vi "NIIE_DoubleClick.vi"(7 "Fill Color":T7=16860, 8 "Error":errorcluster, 9 "Data":T1={"Class"={"Ants"=refnum, "Layer"=refnum, "Templates"=refnum, "Icon"=refnum, "Glyph"=refnum, "Settings"=refnum, "Tools"=refnum}, "Ref"={"Add Layer"=refnum, "Remove Layer"=refnum, "Line Text"=[], "Body Text Spec"=refnum, "DNL_Font"=refnum, "glyph path str"=refnum, "templates path str"=refnum, "Arrow Up"=refnum, "Arrow Down"=refnum, "IE VI Ref"=refnum, "Glyphs tree"=refnum, "Templates tree"=refnum, "Layer Icon Text"=refnum, "Layer Template"=refnum, "Clipboard"=refnum, "BW icon in"=refnum, "Color icon in"=refnum, "Layer Clust"=refnum, "Body Text"=refnum, "DNL_Framework Templates"=refnum, "Search Templates"=refnum, "TextMarker"=refnum, "Tab Control"=refnum, "Search Glyphs"=refnum, "Line Color"=refnum, "DNL_Glyphs []"=refnum, "Fill Color"=refnum, "Tools"=refnum, "Glyphs tree"=refnum, "Icon"=refnum, "Preview"=refnum, "Ants"=refnum, "Terminals"=refnum, "menu reference"=refnum, "LayerNames"=[], "GlyphLoadAnimation"=refnum, "TemplateLoadAnimation"=refnum, "refreshGlyphs"=refnum, "refreshTemplates"=refnum}, "Support"={"AntsRect"={"left"=0, "top"=0, "right"=0, "bottom"=0}, "Mouse Move Coords"={"Horizontal"=0, "Vertical"=0}, "Mouse Down Coords"={"Horizontal"=0, "Vertical"=0}, "Temp Coord"={"Horizontal"=0, "Vertical"=0}, "Action"=enum."Default", "Edge Color"=4914962, "Fill Color"=16860, "Mouse Down?"=FALSE, "Draft Mode?"=FALSE, "Temp Icon"=bytes[3102], "CTRL Pressed"=FALSE, "Move Selection?"=FALSE, "AntsRect Orig"={"left"=0, "top"=0, "right"=0, "bottom"=0}, "Text"="", "TM Set?"=FALSE, "Mouse inside icon?"=FALSE, "Tool (old value)"=0, "Pencil Move Color"=0, "Swap Colors?"=FALSE, "Shift pressed?"=FALSE}}, 11 "Edge Color":T7=16860) -> (0 "Error Out":errorcluster, 1 "Name Out":string, 3 "New Picture Out":picture, 4 "Active Tool Out":T8=enum."Ellipse", 5 "Invalid Picture? Out":bool)   [LabVIEW 2021]
uses:
  vi.lib/LabVIEW Icon API/lv_icon/Controls/IEColor.ctl
  MB CORE/TypeDefs/Cluster_Button Draw Tools.ctl
  MB CORE/TypeDefs/Bool_Draw Tool.ctl
  MB CORE/TypeDefs/Bool_Line Tool.ctl
  MB CORE/TypeDefs/Bool_ColorExtractor Tool.ctl
  MB CORE/TypeDefs/Bool_Fill Tool.ctl
  MB CORE/TypeDefs/Bool_IERect Tool.ctl
  MB CORE/TypeDefs/Bool_FRect Tool.ctl
  MB CORE/TypeDefs/Bool_Circle Tool.ctl
  MB CORE/TypeDefs/Bool_FillCircle Tool.ctl
  MB CORE/TypeDefs/Bool_Eraser Tool.ctl
  MB CORE/TypeDefs/Bool_Text Tool.ctl
  MB CORE/TypeDefs/Bool_Selection Tool.ctl
  MB CORE/TypeDefs/Bool_Move Tool.ctl
  Controls/IE Data.ctl
  Class/Tools/Tools Paint.lvclass
  Class/Ants/Ants.lvclass
  Class/FakedArray/FakedArray.lvclass
  vi.lib/LabVIEW Icon API/lv_icon/Classes/Icon/Icon.lvclass
  Class/Icon Library/Glyph.lvclass
  Class/Settings/Settings.lvclass
  Controls/IE Classes.ctl
  Controls/References Cluster.ctl
  Controls/SupportClass.ctl
  <vilib>/Utility/miscctls.llb/LVPoint32TypeDef.ctl
  Controls/ENUM_SupportClass_Action.ctl
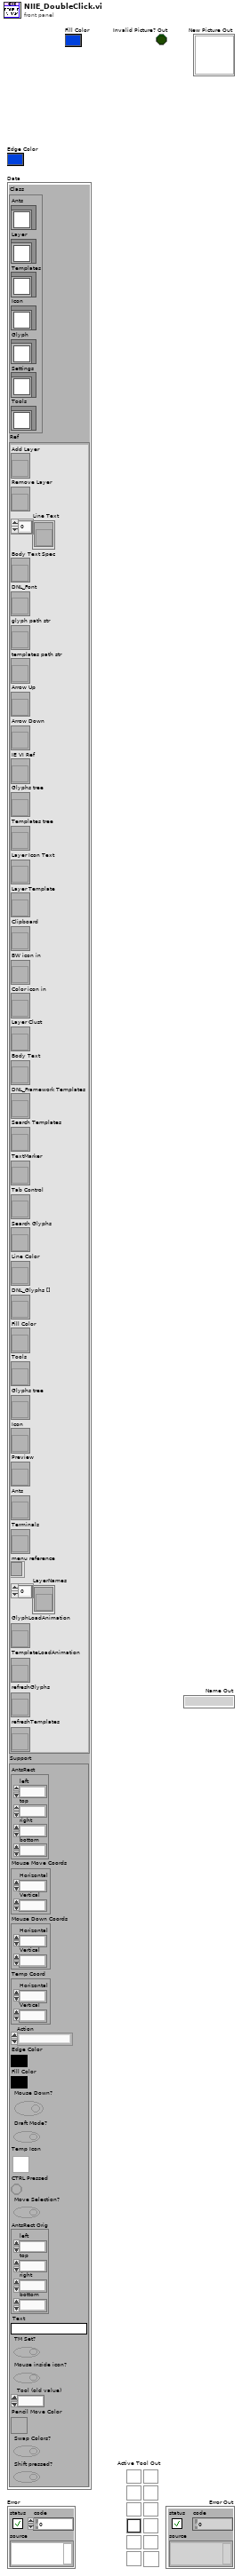
[diagram p1: front panel]
types:
  T1 = typedef "IE Data.ctl" = cluster{"Class":T2, "Ref":T3, "Support":T4}
  T2 = typedef "IE Classes.ctl" = cluster{"Ants":refnum<class "Ants.lvclass">, "Layer":refnum<class "FakedArray.lvclass">, "Templates":refnum<class "FakedArray.lvclass">, "Icon":refnum<class "Icon.lvclass">, "Glyph":refnum<class "Glyph.lvclass">, "Settings":refnum<class "Settings.lvclass">, "Tools":refnum<class "Tools Paint.lvclass">}
  T3 = typedef "References Cluster.ctl" = cluster{"Add Layer":refnum<vi>, "Remove Layer":refnum<vi>, "Line Text":refnum<vi>[], "Body Text Spec":refnum<vi>, "DNL_Font":refnum<vi>, "glyph path str":refnum<vi>, "templates path str":refnum<vi>, "Arrow Up":refnum<vi>, "Arrow Down":refnum<vi>, "IE VI Ref":refnum<vi>, "Glyphs tree":refnum<vi>, "Templates tree":refnum<vi>, "Layer Icon Text":refnum<vi>, "Layer Template":refnum<vi>, "Clipboard":refnum<vi>, "BW icon in":refnum<vi>, "Color icon in":refnum<vi>, "Layer Clust":refnum<vi>, "Body Text":refnum<vi>, "DNL_Framework Templates":refnum<vi>, "Search Templates":refnum<vi>, "TextMarker":refnum<vi>, "Tab Control":refnum<vi>, "Search Glyphs":refnum<vi>, "Line Color":refnum<vi>, "DNL_Glyphs []":refnum<vi>, "Fill Color":refnum<vi>, "Tools":refnum<vi>, "Glyphs tree":refnum<vi>, "Icon":refnum<vi>, "Preview":refnum<vi>, "Ants":refnum<vi>, "Terminals":refnum<vi>, "menu reference":refnum<k9>, "LayerNames":refnum<vi>[], "GlyphLoadAnimation":refnum<vi>, "TemplateLoadAnimation":refnum<vi>, "refreshGlyphs":refnum<vi>, "refreshTemplates":refnum<vi>}
  T4 = typedef "SupportClass.ctl" = cluster{"AntsRect":cluster{"left":i16, "top":i16, "right":i16, "bottom":i16}, "Mouse Move Coords":T5, "Mouse Down Coords":T5, "Temp Coord":T5, "Action":T6, "Edge Color":T7, "Fill Color":T7, "Mouse Down?":bool, "Draft Mode?":bool, "Temp Icon":picture, "CTRL Pressed":bool, "Move Selection?":bool, "AntsRect Orig":cluster{"left":i16, "top":i16, "right":i16, "bottom":i16}, "Text":string, "TM Set?":bool, "Mouse inside icon?":bool, "Tool (old value)":u32, "Pencil Move Color":u32, "Swap Colors?":bool, "Shift pressed?":bool}
  T5 = typedef "LVPoint32TypeDef.ctl" = cluster{"Horizontal":i32, "Vertical":i32}
  T6 = typedef "ENUM_SupportClass_Action.ctl" = enum16{"Default", "Move Selection", "Glyph Library", "Tool"}
  T7 = typedef "IEColor.ctl" = u32
  T8 = typedef "Cluster_Button Draw Tools.ctl" = enum32{"Pencil", "Line", "Dropper", "Fill", "Rectangle", "Filled Rectangle", "Ellipse", "Filled Ellipse", "Eraser", "Text", "Select", "Move"}
  T9 = cluster{"left":i16, "top":i16, "right":i16, "bottom":i16}
  T10 = cluster{"Left":i32, "Top":i32, "Right":i32, "Bottom":i32}
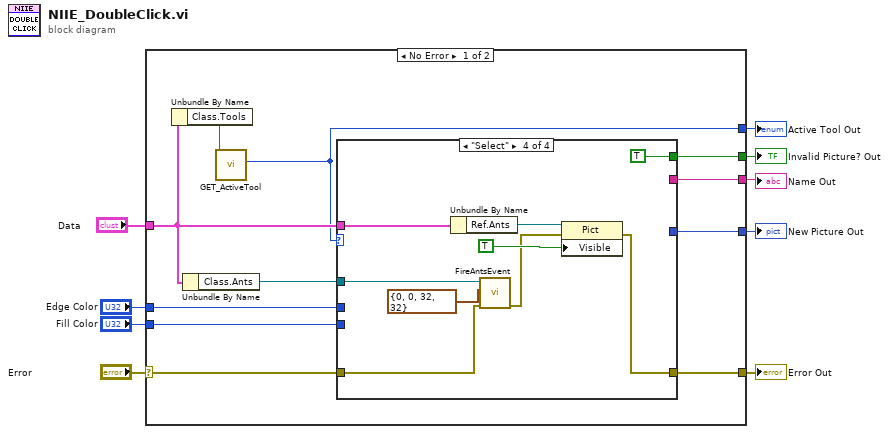
[diagram p0: block diagram]
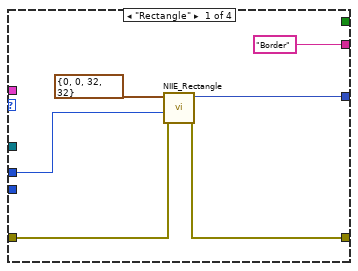
[diagram p2: hidden frame]
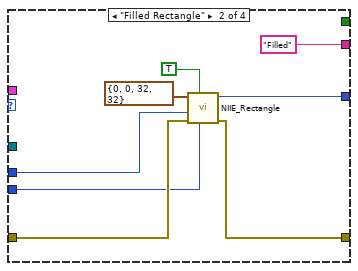
[diagram p3: hidden frame]
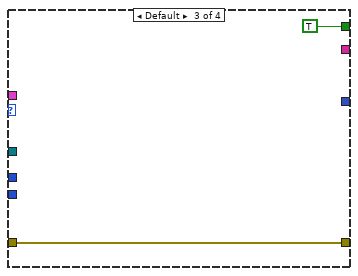
[diagram p4: hidden frame]
diagram:
  n1 = case shown="No Error" "Error" {
    selector: "Error" -> [w19 w46]
    tunnel: [w18 w46] -> w8
    tunnel: "Edge Color" -> [w20 _]
    tunnel: [w17 _] -> w6
    tunnel: [w16 _] -> w5
    tunnel: [w15 _] -> w4
    tunnel: [w10 _] -> w3
    tunnel: "Fill Color" -> [w14 _]
    tunnel: "Data" -> [w12 _]
    frame No Error {
      n2 = Unbundle By Name(w12) -> ("Class.Tools"=w11:refnum<class "Tools Paint.lvclass">)
      n3 = Unbundle By Name(w12) -> ("Class.Ants"=w13:refnum<class "Ants.lvclass">)
      n4 = call-dynamic "GET_ActiveTool.vi"("Tools Paint.lvclass in"=w11) -> ("Radio Buttons"=w10:T8)  [unwired: 8 in, 2 out]
      n5 = case shown="\"Select\"" w10 {
        tunnel: w20 -> [w26 w34 _ _]
        tunnel: w19 -> [w25 w33 w36 w37]
        tunnel: [w24 w32 w36 w39] -> w18
        tunnel: [w21 w27 _ _] -> w17
        tunnel: [_ _ TRUE TRUE] -> w16
        tunnel: ["Border" ("String 2") "Filled" ("String") _ _] -> w15
        tunnel: w13 -> [_ _ _ w44]
        tunnel: w14 -> [_ w29 _ _]
        tunnel: w12 -> [_ _ _ w38]
        frame "Rectangle" {
          n6 = call "NIIE_Rectangle.vi"("Error"=w25, "Edge Color"=w26, "Rect"=T9 {"left"=0, "top"=0, "right"=32, "bottom"=32} ("rect")) -> ("Error Out"=w24:errorcluster, "New Picture Out"=w21:picture)  [unwired: 7 in]
        }
        frame "Filled Rectangle" {
          n7 = call "NIIE_Rectangle.vi"("Fill Color"=w29, "Fill?(F)"=TRUE ("fill?(F)"), "Error"=w33, "Edge Color"=w34, "Rect"=T9 {"left"=0, "top"=0, "right"=32, "bottom"=32} ("rect")) -> ("Error Out"=w32:errorcluster, "New Picture Out"=w27:picture)  [unwired: 5 in]
        }
        frame Default {
        }
        frame "Select" {
          n8 = Unbundle By Name(w38) -> ("Ref.Ants"=w42:refnum<vi>)
          n9 = call "FireAntsEvent.vi"("error in (no error)"=w37, "Rectangle (default: deselect)"=T10 {"Left"=0, "Top"=0, "Right"=32, "Bottom"=32} ("Rectangle"), "Ants in"=w44) -> ("error out"=w40:errorcluster)  [unwired: 1 in, 7 out]
          n10 = property class="Pict"(reference=w42, error in=w40, "Visible"=TRUE) -> (error out=w39:errorcluster)  [unwired: 1 out]
        }
      }
    }
    frame Error {
    }
  }
  "Error Out" <- w8
  "New Picture Out" <- w6
  "Name Out" <- w4
  "Invalid Picture? Out" <- w5
  "Active Tool Out" <- w3
